vi "Siargo Mass Flow Meter Example.vi"() -> ()   [LabVIEW 2020]
uses:
  Controls/Siargo Main Control.ctl
panel:
  out "error out 2":errorcluster
  in  "error in (no error)":errorcluster
  out "Siargo Control Output":T1
  in  "VISA resource name":refnum<visa-resource-name>
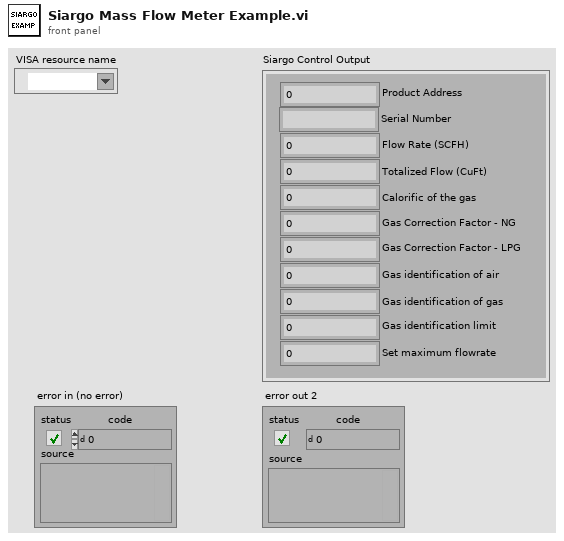
[diagram p1: front panel]
types:
  T1 = typedef "Siargo Main Control.ctl" = cluster{"Flow Rate (SCFH)":dbl, "Totalized Flow (CuFt)":dbl, "Product Address":u16, "Calorific of the gas":u16, "Gas Correction Factor - NG":u16, "Gas Correction Factor - LPG":u16, "Gas identification of air":u16, "Gas identification of gas":u16, "Gas identification limit":u16, "Set maximum flowrate":dbl, "Serial Number":string}
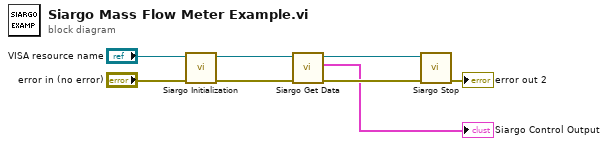
[diagram p0: block diagram]
diagram:
  n1 = call "Siargo Initialization.vi"("error in (no error)"="error in (no error)", "VISA resource name"="VISA resource name") -> ("error out"=w5:errorcluster, "serial master instance"=w8:refnum<class "Modbus Master.lvclass">)  [unwired: 8 in]
  n2 = call "Siargo Get Data.vi"("error in"=w5, "serial master instance"=w8) -> ("error out"=w6:errorcluster, "Siargo Control Output"=→"Siargo Control Output":T1, "Modbus API out"=w7:refnum<class "Modbus Master.lvclass">)  [unwired: 7 in]
  n3 = call "Siargo Stop.vi"("error in"=w6, "Modbus master in"=w7) -> ("error out"=→"error out 2":errorcluster)  [unwired: 9 in]
